vi "GetEpochTrace.vi"(5 "File Paramters":T2, 6 "Parameters for Optic stimulation":T1, 7 "Whole Trace":sgl[][](graph)) -> (3 "Epoch":sgl[][](graph))   [LabVIEW 2017]
uses:
  Class, Controls/Parameters for Optic Stimulation.ctl
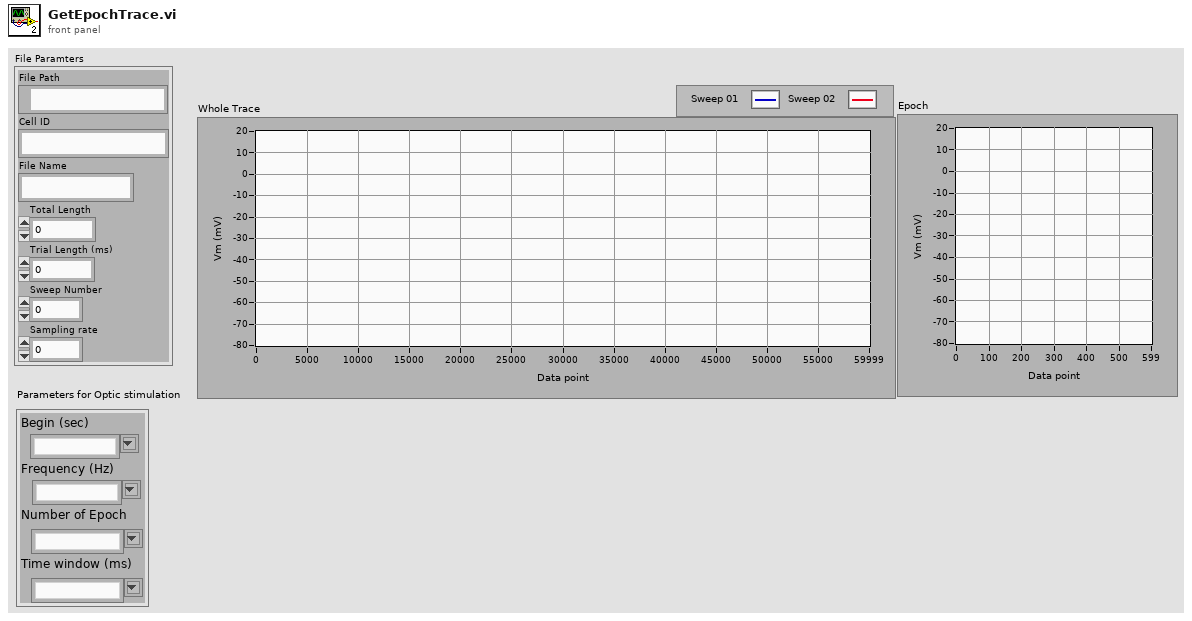
[diagram p1: front panel]
types:
  T1 = typedef "Parameters for Optic Stimulation.ctl" = cluster{"Begin (sec)":string, "Frequency (Hz)":string, "Number of Epoch":string, "Time window (ms)":string}
  T2 = cluster{"File Path":path, "Cell ID":string, "File Name":string, "Total Length":i32, "Trial Length (ms)":dbl, "Sweep Number":dbl, "Sampling rate":dbl}
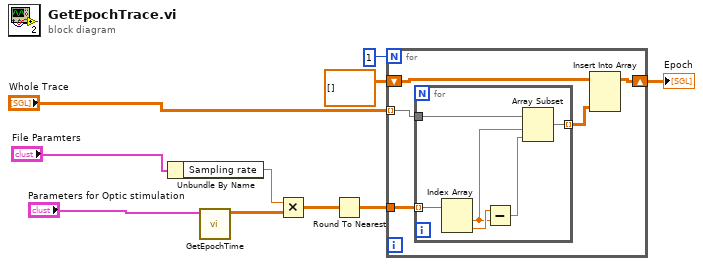
[diagram p0: block diagram]
diagram:
  n1 = Unbundle By Name("File Paramters") -> ("Sampling rate"=w8:dbl)
  n2 = call "GetEpochTime.vi"("Parameters for Optic stimulation"="Parameters for Optic stimulation") -> ("Epoch begin / end"=w7:dbl[][])  [unwired: 6 in]
  n3 = Multiply(x=w8, y=w7) -> (x*y=w6:dbl[][])
  n4 = Round To Nearest(number=w6) -> (nearest integer value=w5:dbl[][])
  n5 = for {
    N: 1 -> [_]
    tunnel: w5 -> [w15]
    tunnel: "Whole Trace" -> [w14] mode=indexing
    shift-right: [w12] -> w2
    shift-left: sgl[][] [] -> [w11]
    n6 = for {
      tunnel: w15 -> [w20] mode=indexing
      tunnel: w14 -> [w21]
      tunnel: [w16] -> w13 mode=indexing
      n7 = Index Array(array=w20) -> (element #1=w18:dbl, element #2=w19:dbl)  [unwired: 2 in]
      n8 = Subtract(x=w19, y=w18) -> (x-y=w17:dbl)
      n9 = Array Subset(array=w21, index=w18, length=w17) -> (w16:sgl[])
    }
    n10 = Insert Into Array(array=w11, new element=w13) -> (w12:sgl[][])  [unwired: 2 in]
  }
  "Epoch" <- w2
